vi "Main.vi"(11 "Module Admin":refnum<class "Delacor_lib_QMH_Module Admin.lvclass">) -> ()   [LabVIEW 2020, in "TCP Server.lvlib"]
doc: "This template is based off of the Queued Message Handler design pattern and the Queued Message Handler project template that ships with LabVIEW.\n\nThe main difference is that the queue is private to this module and communication between modules is performed via Broadcast and Request events.\n\nRequest events are wrapped in public API methods and are handled in the Event Handling Loop (EHL) of this VI. Any module can register for Broadcast events sent by this module. The EHL generates messages based on user interface actions.\n\nThe Message Handling Loop (MHL) processes messages generated by the EHL, or by other messages. The messages are string values, so new messages can be added easily to the Message Cases case structure in the MHL. Each message cluster can also provide an optional value for Message Data, which is a variant that can be converted to whatever message-specific data is required.\n_____\nBased on DQMH Project Template 6.0.0.91."
uses:
  TCP Server.lvlib
  <vilib>/Delacor/Delacor QMH/Libraries/Module Admin_class/Delacor_lib_QMH_Module Admin.lvclass
  Module Data--cluster.ctl
  <vilib>/Delacor/Delacor QMH/Libraries/Message Queue_class/Delacor_lib_QMH_Message Queue.lvclass/Delacor_lib_QMH_Message Queue.ctl
  Stop Argument--cluster.ctl
  <vilib>/Delacor/Delacor QMH/Libraries/Module Admin_class/Delacor_lib_QMH_Module Admin.lvclass/Delacor_lib_QMH_Module Admin.ctl
  <vilib>/Utility/miscctls.llb/LVPointTypeDef.ctl
  <vilib>/Delacor/Delacor QMH/Libraries/Message Queue_class/Delacor_lib_QMH_Enqueue Message (Single).vi
  <vilib>/Delacor/Delacor QMH/Libraries/Module Admin_class/Delacor_lib_QMH_Get External Launch.vi
  <vilib>/Utility/error.llb/Error Cluster From Error Code.vi
  <vilib>/ErrorRing/Error Ring.xnode
  <vilib>/Delacor/Delacor QMH/Libraries/Message Queue_class/Delacor_lib_QMH_Message Queue.lvclass
  TCP Client/TCP Client.lvlib
panel:
  in  "Numeric":i32=-1
  out "Ring":i32(ring) items=["All"=-1]
  in  "DATA":cluster{"Slide":dbl, "Knob":dbl, "Boolean":bool} {"Knob" scale=0.0..10.0; "Slide" scale=0.0..10.0}
  out "# of Connections":i32
  out "error out":errorcluster
  out "Status":string
  in  "Simulate MHL Error":bool
  in  "Simulate EHL Error":bool
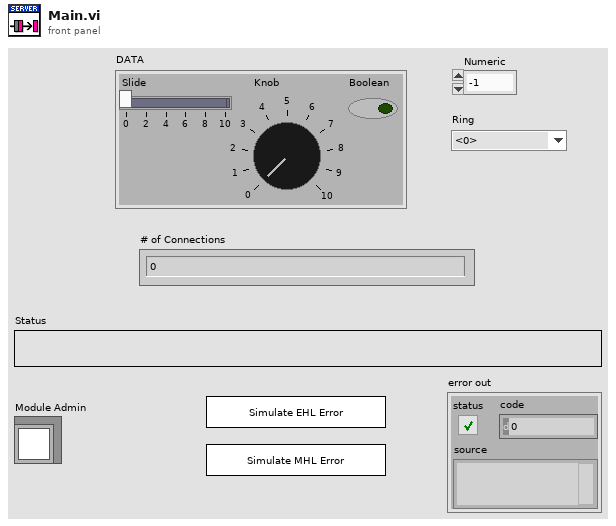
[diagram p1: front panel]
types:
  T1 = typedef "TCP Server.lvlib/Request Events--cluster.ctl" = cluster{"Stop Module":refnum<user-event>, "Show Panel":refnum<user-event>, "Hide Panel":refnum<user-event>, "Get Module Execution Status":refnum<user-event>, "Show Diagram":refnum<user-event>, "Wake Up Helper Loop":refnum<user-event>}
  T2 = typedef "TCP Client.lvlib/Broadcast Events--cluster.ctl" = cluster{"Module Did Init":refnum<user-event>, "Status Updated":refnum<user-event>, "Error Reported":refnum<user-event>, "Module Did Stop":refnum<user-event>, "Update Module Execution Status":refnum<user-event>}
  T3 = typedef "TCP Server.lvlib/Module Data--cluster.ctl" = cluster{"Status":string, "listener":refnum<k5>}
  T4 = enum32{"invalid lock state", "Not Locked", "Locked (No Password)", "Password-protected"}
  T5 = typedef "TCP Server.lvlib/Stop Argument--cluster.ctl" = cluster{"Origin":string, "Exit via Stop Module Req?":bool, "Wait for Module to stop?":bool}
  T6 = typedef "LVPointTypeDef.ctl" = cluster{"Horizontal":i16, "Vertical":i16}
  T7 = enum32{"Invalid", "Standard", "Closed", "Hidden", "Minimized", "Maximized"}
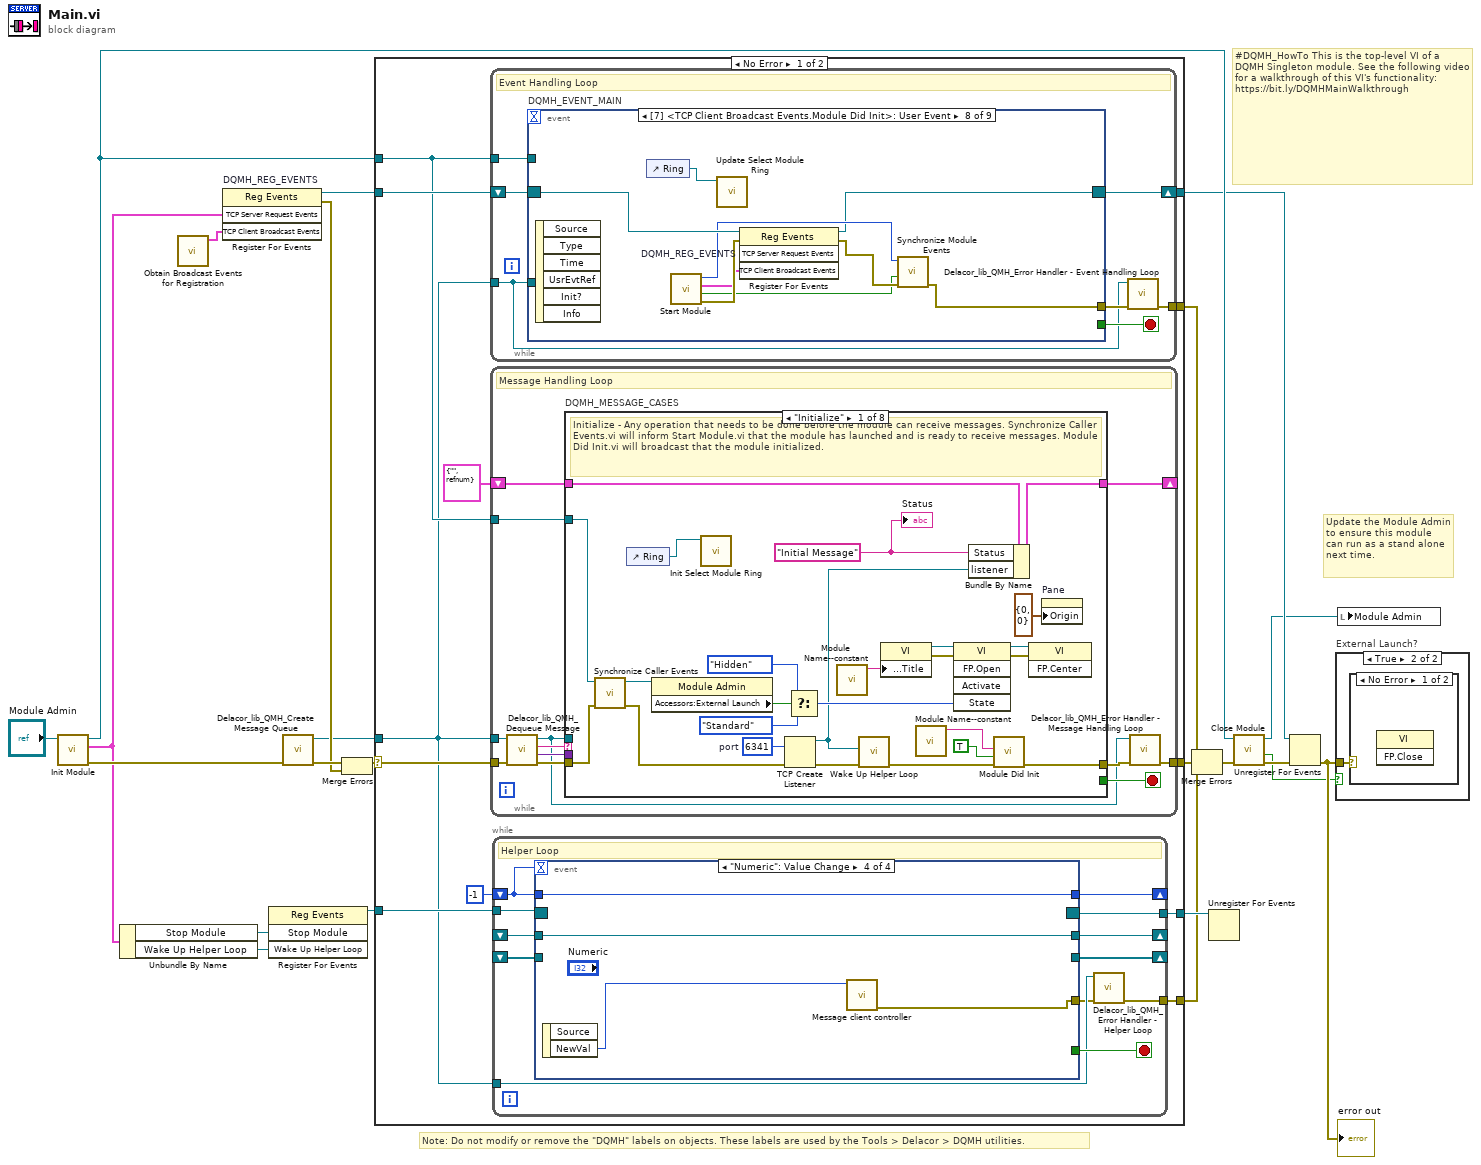
[diagram p0: block diagram]
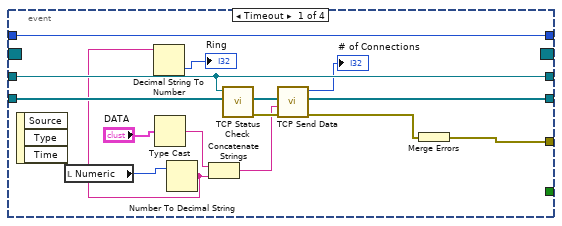
[diagram p2: hidden frame]
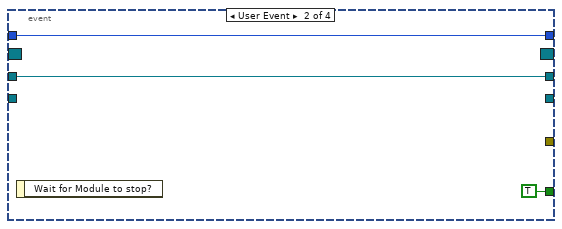
[diagram p3: hidden frame]
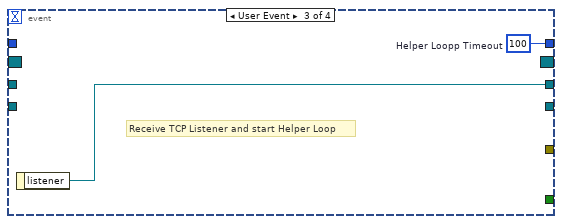
[diagram p4: hidden frame]
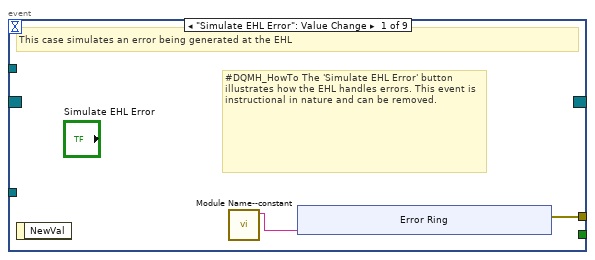
[diagram p5: hidden frame]
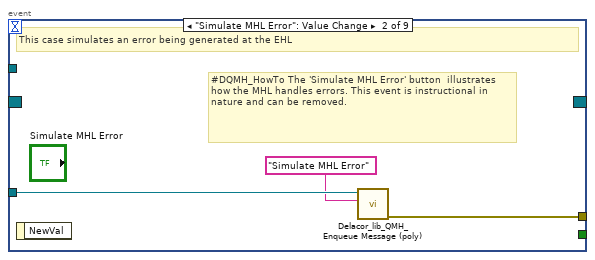
[diagram p6: hidden frame]
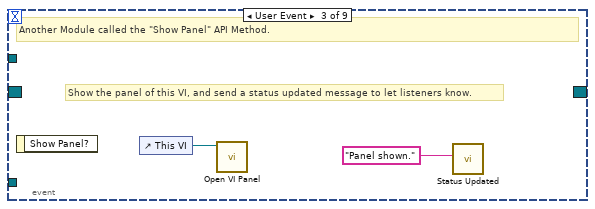
[diagram p7: hidden frame]
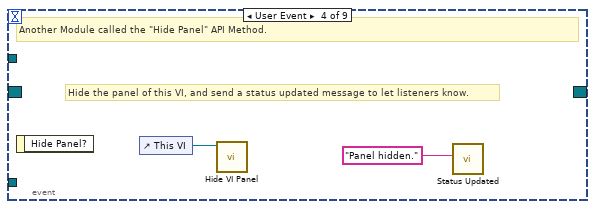
[diagram p8: hidden frame]
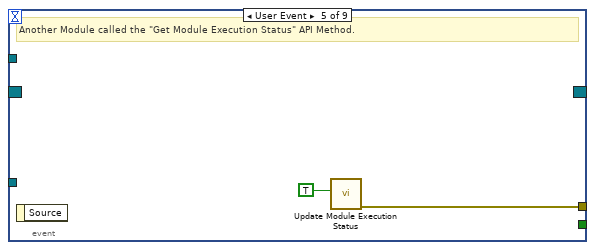
[diagram p9: hidden frame]
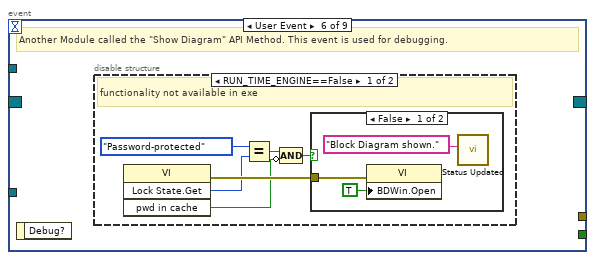
[diagram p10: hidden frame]
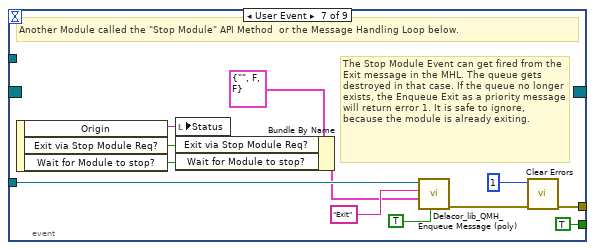
[diagram p13: hidden frame]
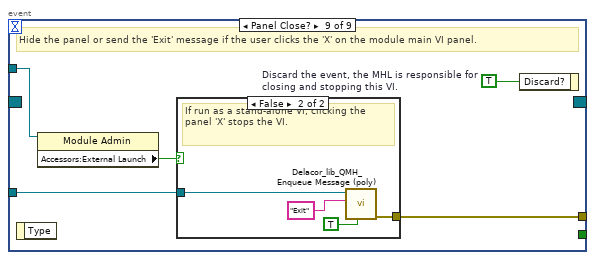
[diagram p14: hidden frame]
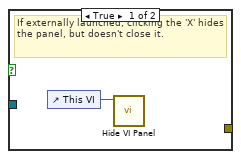
[diagram p15: hidden frame]
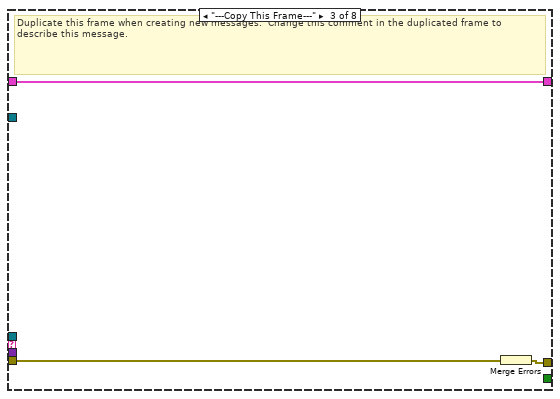
[diagram p17: hidden frame]
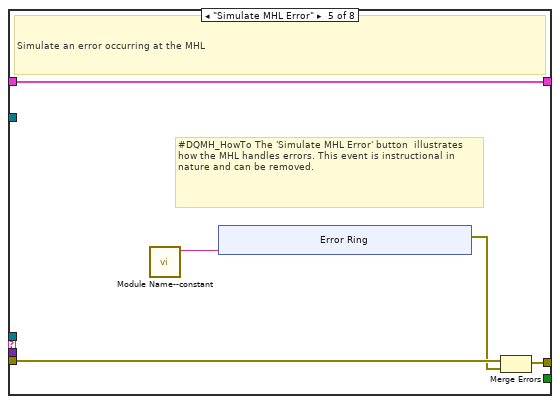
[diagram p19: hidden frame]
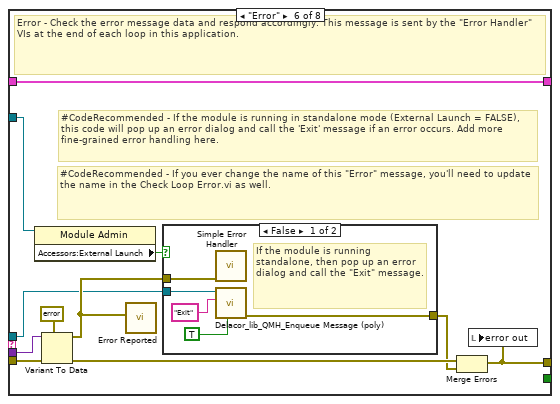
[diagram p20: hidden frame]
diagram:
  # "#DQMH_HowTo This is the top-level VI of a DQMH Singleton module. See the following video for a walkthrough of this VI's functionality: https://bit.ly/DQMHMainWalkthrough"
  # "Note: Do not modify or remove the \"DQMH\" labels on objects. These labels are used by the Tools > Delacor > DQMH utilities."
  # "Update the Module Admin to ensure this module can run as a stand alone next time."
  n1 = call "Init Module.vi"("Singleton Module Admin in"="Module Admin") -> ("error out"=w22:errorcluster, "TCP Server Request Events"=w6:T1, "Singleton Module Admin out"=w14:refnum<class "Delacor_lib_QMH_Module Admin.lvclass">)  [unwired: 8 in]
  n2 = Unbundle By Name(w6) -> ("Stop Module"=w5:refnum<user-event>, "Wake Up Helper Loop"=w2:refnum<user-event>)
  n3 = call "Obtain Broadcast Events for Registration.vi"() -> ("TCP Client Broadcast Events"=w1:T2)  [unwired: 9 in, 2 out]
  n4 = register-events "DQMH_REG_EVENTS"(w6, w1) -> (reference out=w12:refnum<event-registration>, error out=w15:errorcluster)  [unwired: 2 in]
  n5 = register-events(w5, w2) -> (reference out=w7:refnum<event-registration>)  [unwired: 2 in, 1 out]
  n6 = call <vilib>:"Delacor_lib_QMH_Create Message Queue.vi"("error in"=w22) -> ("error out"=w17:errorcluster, "Message Queue"=w11:refnum<class "Delacor_lib_QMH_Message Queue.lvclass">)  [unwired: 9 in]
  n7 = Merge Errors(w17, w15) -> (w16:errorcluster)
  n8 = case shown="No Error" w16 {
    selector: w16 -> [w33 w241]
    tunnel: [w35 w238] -> w23
    tunnel: [w32 w246] -> w13
    tunnel: w12 -> [w30 w246]
    tunnel: w11 -> [w25 w240]
    tunnel: [w34 _] -> w20
    tunnel: w14 -> [w29 w242]
    tunnel: w7 -> [w28 w239]
    tunnel: [w27 w239] -> w4
    tunnel: [w26 w238] -> w3
    frame No Error {
      n9 = while {
        tunnel: w25 -> [w72]
        shift-right: [w75] -> w32
        shift-left: w30 -> [w76]
        tunnel: [w77] -> w34
        tunnel: w29 -> [w73]
        stop <- w74 stop-if-true
        # "Event Handling Loop"
        n10 = event "DQMH_EVENT_MAIN" shown="[7] <TCP Client Broadcast Events.Module Did Init>: User Event" {
          selector: w76 -> [_ _ _ _ _ _ _ w125 _]
          dyn-events: [_ _ _ _ _ _ _ w118 _] -> w75
          timeout: _ -> [_ _ _ _ _ _ _ _ _]
          tunnel: [_ _ _ _ _ _ TRUE ("Discard?") _ _] -> w74
          tunnel: w72 -> [_ w89 _ _ _ _ w113 _ w129]
          tunnel: [w80 w90 _ _ w96 _ w116 w119 w131] -> w78
          tunnel: w73 -> [_ _ _ _ _ _ _ _ w128]
          event "Simulate EHL Error": Value Change {
            # "#DQMH_HowTo The 'Simulate EHL Error' button  illustrates how the EHL handles errors. This event is instructional in nature and can be removed."
            # "This case simulates an error being generated at the EHL"
            n11 = event-data() -> ()  [unwired: 1 in, 1 out]
            n12 = call "Module Name--constant.vi"() -> ("Module Name"=w79:string)  [unwired: 11 in]
            n13 = xnode "Error Ring"("parameter 0"=w79) -> ("error out"=w80:errorcluster)
          }
          event "Simulate MHL Error": Value Change {
            # "#DQMH_HowTo The 'Simulate MHL Error' button  illustrates how the MHL handles errors. This event is instructional in nature and can be removed."
            # "This case simulates an error being generated at the EHL"
            n14 = event-data() -> ()  [unwired: 1 in, 1 out]
            n15 = call-poly <vilib>:"Delacor_lib_QMH_Enqueue Message (poly).vi"("Message"="Simulate MHL Error", "Message Queue in"=w89) -> ("error out"=w90:errorcluster)  [unwired: 8 in, 1 out]
          }
          event User Event {
            # "Show the panel of this VI, and send a status updated message to let listeners know."
            # "Another Module called the \"Show Panel\" API Method."
            n16 = event-data() -> ()  [unwired: 1 in, 1 out]
            n17 = control-ref of="This VI"() -> (w92:refnum<vi>)
            n18 = call "Open VI Panel.vi"("VI"=w92) -> ()  [unwired: 10 in, 1 out]
            n19 = call "Status Updated.vi"("Status"="Panel shown." ("format string")) -> ()  [unwired: 10 in, 1 out]
          }
          event User Event {
            # "Hide the panel of this VI, and send a status updated message to let listeners know."
            # "Another Module called the \"Hide Panel\" API Method."
            n20 = event-data() -> ()  [unwired: 1 in, 1 out]
            n21 = control-ref of="This VI"() -> (w94:refnum<vi>)
            n22 = call "Hide VI Panel.vi"("VI"=w94) -> ()  [unwired: 10 in, 1 out]
            n23 = call "Status Updated.vi"("Status"="Panel hidden." ("format string")) -> ()  [unwired: 10 in, 1 out]
          }
          event User Event {
            # "Another Module called the \"Get Module Execution Status\" API Method."
            n24 = event-data() -> ()  [unwired: 1 in, 1 out]
            n25 = call "Update Module Execution Status.vi"("Running?"=TRUE) -> ("error out"=w96:errorcluster)  [unwired: 10 in]
          }
          event User Event {
            # "Another Module called the \"Show Diagram\" API Method. This event is used for debugging."
            n26 = event-data() -> ()  [unwired: 1 in, 1 out]
            n27 = disable-structure shown="RUN_TIME_ENGINE==False" {
              frame condition #0 (active) {
                # "functionality not available in exe"
                n28 = invoke class="VI" method="Lock State.Get"() -> (error out=w102:errorcluster, "Get Lock State"=w101:T4, "pwd in cache"=w98:bool)  [unwired: 4 in, 1 out]
                n29 = Equal?(x=T4."Password-protected", y=w101) -> (x = y?=w99:bool)
                n30 = Compound Arithmetic op=AND(w99, invert w98) -> (w97:bool)
                n31 = case shown="False" w97 {
                  tunnel: w102 -> [w105 _]
                  frame False {
                    n32 = property class="VI"(error in=w105, "BDWin.Open"=TRUE ("Block Diagram Window:Open")) -> ()  [unwired: 1 in, 2 out]
                    n33 = call "Status Updated.vi"("Status"="Block Diagram shown." ("format string")) -> ()  [unwired: 10 in, 1 out]
                  }
                  frame True {
                    # "Password-protected VI, and the password is not in the cache. Do not show the diagram."
                  }
                }
              }
              frame condition #1 {
              }
            }
          }
          event User Event {
            # "The Stop Module Event can get fired from the Exit message in the MHL. The queue gets destroyed in that case. If the queue no longer exists, the Enqueue Exit as a priority message will return error 1. It is safe to ignore, because the module is already exiting."
            # "Another Module called the \"Stop Module\" API Method  or the Message Handling Loop below."
            n34 = event-data() -> ("Origin"=w112:string, "Exit via Stop Module Req?"=w108:bool, "Wait for Module to stop?"=w107:bool)  [unwired: 1 in]
            n35 = local write "Status"(w112) -> ()
            n36 = Bundle By Name(cluster=T5 {"Origin"="", "Exit via Stop Module Req?"=FALSE, "Wait for Module to stop?"=FALSE} ("Stop Argument"), "Exit via Stop Module Req?"=w108, "Wait for Module to stop?"=w107) -> (w106:T5)
            n37 = call-poly <vilib>:"Delacor_lib_QMH_Enqueue Message (poly).vi"("Priority Message? (F)"=TRUE, "Message Data"=w106, "Message"="Exit", "Message Queue in"=w113) -> ("error out"=w117:errorcluster)  [unwired: 6 in, 1 out]
            n38 = call <vilib>:"Clear Errors.vi"("error in (no error)"=w117, "specific error code to clear (0: all)"=1) -> ("error out"=w116:errorcluster)  [unwired: 4 in, 1 out]
          }
          event User Event {
            n39 = event-data() -> ()  [unwired: 1 in, 6 out]
            n40 = control-ref of="Ring"() -> (w126:refnum<vi>)
            n41 = call "Start Module.vi"() -> ("error out"=w124:errorcluster, "Wait for Event Sync?"=w122:bool, "TCP Client Broadcast Events"=w120:T2, "Module ID"=w121:i32)  [unwired: 8 in]
            n42 = call "Update Select Module Ring.vi"("Select Module Ring Ref"=w126) -> ()  [unwired: 8 in, 3 out]
            n43 = register-events "DQMH_REG_EVENTS"(reference=w125, error in=w124, w120) -> (reference out=w118:refnum<event-registration>, error out=w123:errorcluster)  [unwired: 1 in]
            n44 = call "Synchronize Module Events.vi"("error in"=w123, "Wait for Event Sync?"=w122, "Module ID in"=w121) -> ("error out"=w119:errorcluster)  [unwired: 7 in, 1 out]
          }
          event Panel Close? {
            w130 = TRUE  # Discard the event, the MHL is responsible for closing and stopping this VI.
            # "Hide the panel or send the 'Exit' message if the user clicks the 'X' on the module main VI panel."
            n45 = event-data() -> ()  [unwired: 1 in, 1 out]
            n46 = property class="Module Admin"(reference=w128) -> ("Accessors:External Launch"=w127:bool)  [unwired: 1 in, 2 out]
            n47 = case shown="False" w127 {
              tunnel: w129 -> [_ w135]
              tunnel: [_ w136] -> w131
              frame True {
                # "If externally launched, clicking the 'X' hides the panel, but doesn't close it."
                n48 = control-ref of="This VI"() -> (w132:refnum<vi>)
                n49 = call "Hide VI Panel.vi"("VI"=w132) -> ()  [unwired: 10 in, 1 out]
              }
              frame False {
                # "If run as a stand-alone VI, clicking the panel 'X' stops the VI."
                n50 = call-poly <vilib>:"Delacor_lib_QMH_Enqueue Message (poly).vi"("Priority Message? (F)"=TRUE, "Message"="Exit", "Message Queue in"=w135) -> ("error out"=w136:errorcluster)  [unwired: 7 in, 1 out]
              }
            }
            n51 = event-data("Discard?"=w130) -> ()  [unwired: 1 in, 1 out]
          }
        }
        n52 = call-dynamic "Delacor_lib_QMH_Error Handler - Event Handling Loop.vi"("error in"=w78, "Message Queue in"=w72) -> ("dup error in"=w77:errorcluster)  [unwired: 8 in, 1 out]
      }
      n53 = while {
        tunnel: w25 -> [w139]
        shift-right: [w143] -> _
        shift-left: T3 {"Status"="", "listener"=refnum} ("Data Cluster") -> [w144]
        tunnel: w33 -> [w147]
        tunnel: [w145] -> w35
        tunnel: w29 -> [w137]
        stop <- w142 stop-if-true
        # "Message Handling Loop"
        n54 = call-dynamic "Delacor_lib_QMH_Dequeue Message.vi"("error in"=w147, "Message Queue in"=w139) -> ("error out"=w146:errorcluster, "Message Data"=w140:variant, "Message"=w141:string, "Message Queue out"=w138:refnum<class "Delacor_lib_QMH_Message Queue.lvclass">)  [unwired: 6 in]
        n55 = case "DQMH_MESSAGE_CASES" shown="\"Initialize\"" w141 {
          selector: w141 -> [_ _ _ _ _ _ _ w225]
          tunnel: w138 -> [_ _ _ _ _ w195 w217 _]
          tunnel: w146 -> [w171 w175 w178 w180 w185 w202 w223 w227]
          tunnel: [w170 w175 w177 w180 w184 w198 w220 w228] -> w148
          tunnel: w144 -> [w161 w174 w176 w179 w182 w197 w216 w226]
          tunnel: [w160 w174 w176 w179 w182 w197 w216 w226] -> w143
          tunnel: [_ _ _ _ _ _ w215 _] -> w142
          tunnel: w140 -> [_ _ _ _ _ w196 w214 _]
          tunnel: w137 -> [w162 _ _ _ _ w194 w209 _]
          frame "Initialize" {
            w154 = u16 6341  # port
            w156 = "Initial Message" ("Initial Message")
            # "Initialize - Any operation that needs to be done before the module can receive messages. Synchronize Caller Events.vi will inform Start Module.vi that the module has launched and is ready to receive messages. Module Did Init.vi will broadcast that the module initialized."
            n56 = call "Synchronize Caller Events.vi"("error in (no error)"=w171, "Singleton Module Admin in"=w162) -> ("error out"=w153:errorcluster, "Singleton Module Admin out"=w157:refnum<class "Delacor_lib_QMH_Module Admin.lvclass">)  [unwired: 8 in]
            n57 = control-ref of="Ring"() -> (w149:refnum<vi>)
            n58 = property class="Module Admin"(reference=w157) -> ("Accessors:External Launch"=w166:bool)  [unwired: 1 in, 2 out]
            n59 = call "Init Select Module Ring.vi"("Select Module Ring Ref"=w149) -> ()  [unwired: 8 in, 3 out]
            n60 = TCP Create Listener(8:w153, 10:w154) -> (0:w152:errorcluster, 3:w150:refnum<k5>)  [unwired: 4 out]
            n61 = Select(t=T7."Hidden" ("State"), s=w166, f=T7."Standard" ("State")) -> (s? t:f=w163:T7)
            n62 = call "Module Name--constant.vi"() -> ("Module Name"=w169:string)  [unwired: 11 in]
            n63 = call "Wake Up Helper Loop.vi"("error in"=w152, "listener"=w150) -> ("error out"=w151:errorcluster)  [unwired: 9 in]
            n64 = property class="VI"("Front Panel.Title"=w169) -> (reference out=w168:refnum<vi>, error out=w173:errorcluster)  [unwired: 2 in]
            n65 = call "Module Name--constant.vi"() -> ("Module Name"=w158:string)  [unwired: 11 in]
            n66 = invoke class="VI" method="FP.Open"(reference=w168, error in=w173, "State"=w163) -> (reference out=w167:refnum<vi>, error out=w172:errorcluster)  [unwired: 2 in, 3 out]
            n67 = Bundle By Name(cluster=w161, "Status"=w156, "listener"=w150) -> (w160:T3)
            n68 = call "Module Did Init.vi"("error in (no error)"=w151, "Initialized?"=TRUE, "Origin"=w158) -> ("error out"=w170:errorcluster)  [unwired: 8 in]
            n69 = invoke class="VI" method="FP.Center"(reference=w167, error in=w172) -> ()  [unwired: 1 in, 3 out]
            n70 = property on="Pane" class="Pane"("Origin"=T6 {"Horizontal"=0, "Vertical"=0}) -> ()  [unwired: 2 in, 2 out]
            "Status" <- w156
          }
          frame "---Module Specific---" {
            # "Separator -- The following cases handle messages specific to this Module."
          }
          frame "---Copy This Frame---" {
            # "Duplicate this frame when creating new messages.  Change this comment in the duplicated frame to describe this message."
            n71 = Merge Errors(w178) -> (w177:errorcluster)
          }
          frame "---Exit and Error Handling---" {
            # "Separator - The following cases handle errors and exit messages."
          }
          frame "Simulate MHL Error" {
            # "#DQMH_HowTo The 'Simulate MHL Error' button  illustrates how the MHL handles errors. This event is instructional in nature and can be removed."
            # "Simulate an error occurring at the MHL"
            n72 = call "Module Name--constant.vi"() -> ("Module Name"=w181:string)  [unwired: 11 in]
            n73 = xnode "Error Ring"("parameter 0"=w181) -> ("error out"=w183:errorcluster)
            n74 = Merge Errors(w185, w183) -> (w184:errorcluster)
          }
          frame "Error" {
            # "#CodeRecommended - If you ever change the name of this \"Error\" message, you'll need to update the name in the Check Loop Error.vi as well."
            # "#CodeRecommended - If the module is running in standalone mode (External Launch = FALSE), this code will pop up an error dialog and call the 'Exit' message if an error occurs. Add more fine-grained error handling here."
            # "Error - Check the error message data and respond accordingly. This message is sent by the \"Error Handler\" VIs at the end of each loop in this application."
            n75 = property class="Module Admin"(reference=w194) -> ("Accessors:External Launch"=w193:bool)  [unwired: 1 in, 2 out]
            n76 = Variant To Data(error in=w202, type=errorcluster {"status"=FALSE, "code"=0, "source"=""} ("error constant"), Variant=w196) -> (data=w203:errorcluster, error out=w200:errorcluster)
            n77 = call "Error Reported.vi"("Error"=w203) -> ()  [unwired: 10 in, 1 out]
            n78 = case shown="False" w193 {
              tunnel: [w208 _] -> w199
              tunnel: w195 -> [w206 _]
              tunnel: w203 -> [w207 _]
              frame False {
                # "If the module is running standalone, then pop up an error dialog and call the \"Exit\" message."
                n79 = call <vilib>:"Simple Error Handler.vi"("error in (no error)"=w207) -> ()  [unwired: 4 in, 5 out]
                n80 = call-poly <vilib>:"Delacor_lib_QMH_Enqueue Message (poly).vi"("Priority Message? (F)"=TRUE, "Message"="Exit", "Message Queue in"=w206) -> ("error out"=w208:errorcluster)  [unwired: 7 in, 1 out]
              }
              frame True {
                # "If the module was launched externally, calling the Error Reported broadcast VI is the only action performed by the \"Error\" message. The module's caller can then process the error appropriately."
              }
            }
            n81 = Merge Errors(w200, w199) -> (w198:errorcluster)
            n82 = local write "error out"(w198) -> ()
          }
          frame "Exit" {
            w213 = 91  # 91: not all Exit messages will have an argument
            w215 = TRUE  # Stop the VI
            # "Release the message queue reference"
            # "#CodeNeeded - Add any required cleanup code here"
            # "Exit - Exit the application."
            n83 = Variant To Data(error in=w223, type=T5 {"Origin"="", "Exit via Stop Module Req?"=FALSE, "Wait for Module to stop?"=FALSE} ("Stop Argument"), Variant=w214) -> (data=w211:T5, error out=w219:errorcluster)
            n84 = call <vilib>:"Clear Errors.vi"("error in (no error)"=w219, "specific error code to clear (0: all)"=w213) -> ("error out"=w222:errorcluster)  [unwired: 4 in, 1 out]
            n85 = control-ref of="This VI"() -> (w210:refnum<vi>)
            n86 = call-dynamic "Delacor_lib_QMH_Release Message Queue.vi"("error in"=w222, "Message Queue"=w217) -> ("error out"=w221:errorcluster)  [unwired: 9 in]
            n87 = call "Handle Exit.vi"("Stop Argument"=w211, "Admin in"=w209, "VI reference"=w210) -> ("error out"=w218:errorcluster)  [unwired: 7 in, 1 out]
            n88 = Merge Errors(w221, w218) -> (w220:errorcluster)
          }
          frame Default {
            # "'Default' case only runs if there is a message that isn't defined in any of the other cases.  Output a programming error."
            n89 = call "Module Name--constant.vi"() -> ("Module Name"=w224:string)  [unwired: 11 in]
            n90 = xnode "Error Ring"("parameter 0"=w225, "parameter 1"=w224) -> ("error out"=w229:errorcluster)
            n91 = Merge Errors(w227, w229) -> (w228:errorcluster)
          }
        }
        n92 = call-dynamic "Delacor_lib_QMH_Error Handler - Message Handling Loop.vi"("error in"=w148, "Message Queue in"=w138) -> ("dup error in"=w145:errorcluster)  [unwired: 8 in, 1 out]
      }
      n93 = while {
        tunnel: w28 -> [w47]
        tunnel: [w45] -> w27
        tunnel: [w44] -> w26
        tunnel: w25 -> [w43]
        shift-right: [w42] -> _
        shift-left: _ -> [w41]
        shift-right: [w40] -> _
        shift-left: -1 ("Helper Loopp Timeout") -> [w39]
        shift-right: [w38] -> _
        shift-left: _ -> [w37]
        stop <- w46 stop-if-true
        # "Helper Loop"
        n94 = event shown="[3] \"Numeric\": Value Change" {
          selector: w47 -> [_ _ _ _]
          dyn-events: [_ _ _ _] -> w45
          timeout: w39 -> [_ _ _ _]
          tunnel: [_ TRUE _ _] -> w46
          tunnel: [w61 w64 w67 w71] -> w42
          tunnel: w41 -> [w61 w64 _ w71]
          tunnel: [w62 w63 w66 w70] -> w40
          tunnel: w39 -> [w62 w63 _ w70]
          tunnel: [w59 _ _ _] -> w38
          tunnel: w37 -> [w58 _ _ _]
          tunnel: [w55 _ _ w68] -> w36
          event Timeout {
            n95 = event-data() -> ()  [unwired: 1 in, 3 out]
            n96 = local read "Numeric"() -> (w48:i32)
            n97 = Type Cast(x="DATA") -> (*(type *) &x=w52:string)  [unwired: 1 in]
            n98 = Number To Decimal String(number=w48) -> (decimal integer string=w50:string)  [unwired: 1 in]
            n99 = Decimal String To Number(string=w50) -> (number=→"Ring":i32)  [unwired: 2 in, 1 out]
            n100 = Concatenate Strings(w52, w50) -> (w51:string)
            n101 = call "TCP Status Check.vi"("Clients"=w58, "listener ID in"=w61) -> ("no error"=w57:errorcluster, "Clients"=w60:refnum<k5>[])  [unwired: 7 in, 1 out]
            n102 = call "TCP Send Data.vi"("error out"=w57, "String"=w51, "Clients"=w60) -> ("error out"=w54:errorcluster, "Clients"=w59:refnum<k5>[], "# of Connections"=→"# of Connections":i32)  [unwired: 6 in]
            n103 = Merge Errors(w54) -> (w55:errorcluster)
          }
          event User Event {
            n104 = event-data() -> ()  [unwired: 1 in, 1 out]
          }
          event User Event {
            w66 = 100  # Helper Loopp Timeout
            # "Receive TCP Listener and start Helper Loop"
            n105 = event-data() -> ("listener"=w67:refnum<k5>)  [unwired: 1 in]
          }
          event "Numeric": Value Change {
            n106 = event-data() -> ("NewVal"=w69:i32)  [unwired: 1 in, 1 out]
            n107 = call "Message client controller.vi"("Module ID"=w69) -> ("error out"=w68:errorcluster)  [unwired: 10 in]
          }
        }
        n108 = call-dynamic "Delacor_lib_QMH_Error Handler - Helper Loop.vi"("error in"=w36, "Message Queue in"=w43) -> ("dup error in"=w44:errorcluster)  [unwired: 8 in, 1 out]
      }
    }
    frame Error {
      # "Synchronize Caller Events.vi will inform Start Module.vi that the module has launched and will let the code calling Start Module.vi register for broadcasts and would permit the caller receive the broadcast that an error occurred at launch time."
      n109 = call-dynamic "Delacor_lib_QMH_Release Message Queue.vi"("error in"=w241, "Message Queue"=w240) -> ("error out"=w238:errorcluster)  [unwired: 9 in]
      n110 = call "Synchronize Caller Events.vi"("Singleton Module Admin in"=w242) -> ("error out"=w247:errorcluster)  [unwired: 9 in, 1 out]
      n111 = call "Module Name--constant.vi"() -> ("Module Name"=w245:string)  [unwired: 11 in]
      n112 = Format Into String(format string="An error occurred during initialization. %s is no longer running.", w245) -> (resulting string=w243:string)  [unwired: 2 in, 1 out]
      n113 = Merge Errors(w238, w247) -> (w248:errorcluster)
      n114 = call "Error Reported.vi"("Additional Information"=w243, "Error"=w248) -> ()  [unwired: 9 in, 1 out]
    }
  }
  n115 = Merge Errors(w20, w23, w3) -> (w19:errorcluster)
  n116 = Unregister For Events(event registration refnum=w4) -> ()  [unwired: 1 in, 1 out]
  n117 = call "Close Module.vi"("error in (no error)"=w19, "Module Admin in"=w14) -> ("error out"=w21:errorcluster, "External Launch"=w8:bool, "Module Admin out"=w9:refnum<class "Delacor_lib_QMH_Module Admin.lvclass">)  [unwired: 7 in]
  n118 = Unregister For Events(event registration refnum=w13, error in=w21) -> (error out=w18:errorcluster)
  "error out" <- w18
  n119 = case "External Launch?" shown="True" w8 {
    tunnel: w18 -> [_ w249]
    frame False {
    }
    frame True {
      n120 = case shown="No Error" w249 {
        frame No Error {
          n121 = invoke class="VI" method="FP.Close"() -> ()  [unwired: 3 in, 3 out]
        }
        frame Error {
          n122 = invoke class="VI" method="FP.Open"("Activate"=TRUE ("Activate?")) -> ()  [unwired: 4 in, 5 out]
        }
      }
    }
  }
  n123 = local write "Module Admin"(w9) -> ()
